vi "Remove Multiple Headers.vi"(8 "error in (no error)":errorcluster, 10 "headers (empty: all)":string[](array[string]), 11 "httpHeaders in":refnum<class "httpHeaders.lvclass">) -> (0 "error out":errorcluster, 3 "httpHeaders out":refnum<class "httpHeaders.lvclass">)   [LabVIEW 2020, in "httpClient.lvlib" / "httpHeaders.lvclass"]
uses:
  httpHeaders.lvclass
  httpHeaders.lvclass/httpHeaders.ctl
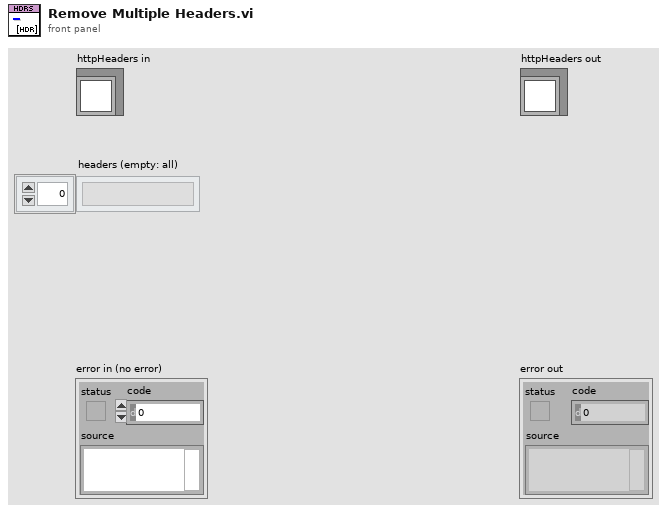
[diagram p1: front panel]
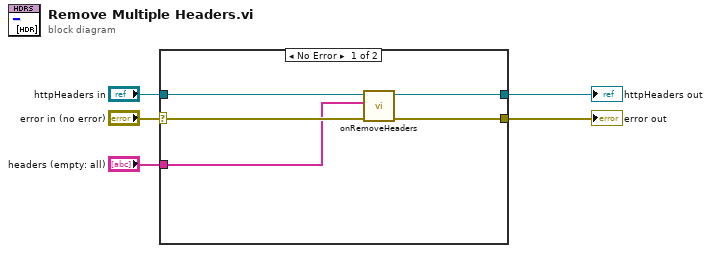
[diagram p0: block diagram]
diagram:
  n1 = case shown="No Error" "error in (no error)" {
    selector: "error in (no error)" -> [w10 w12]
    tunnel: [w9 w12] -> w4
    tunnel: [w8 w11] -> w2
    tunnel: "httpHeaders in" -> [w7 w11]
    tunnel: "headers (empty: all)" -> [w6 _]
    frame No Error {
      n2 = call-dynamic "onRemoveHeaders.vi"("error in (no error)"=w10, "headers (empty: all)"=w6, "httpHeaders in"=w7) -> ("error out"=w9:errorcluster, "httpHeaders out"=w8:refnum<class "httpHeaders.lvclass">)  [unwired: 7 in]
    }
    frame Error {
    }
  }
  "error out" <- w4
  "httpHeaders out" <- w2
